vi "Gen Tophat.vi"(1 "Frequency Span":i32=1, 2 "Lower Frequency \nLocation":i32=4, 3 "Nyquist Frequency\nLocation":i32=16) -> (0 "Waveform Graph":i64[](graph))   [LabVIEW 2015]
doc: "This VI will create the actual frequency domain signal required to generate the top hat signal used for acquiring the resonant frequency. The frequency domain signal will be a signal that will span +/- the Nyquist frequency where the waveform is zero at all values except for +/- the frequencies of interest, where the waveform will be one. \n\nThe reflection of the tophat into the negative frequencies ensures that initially we are genrating a sinusoid in the time domain with only a real component (when sampled however, the signal will have both real and imaginary components, but will still have a tophat like structure in the frequency domain). Ultimately, this VI is used to feed into an IDFT for development of a time domain signal."
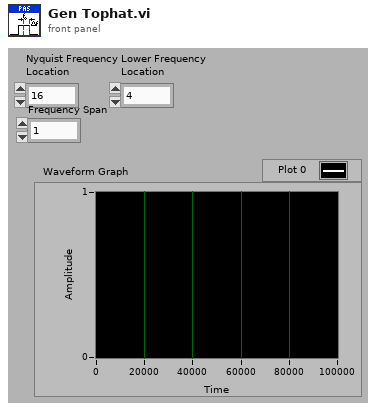
[diagram p1: front panel]
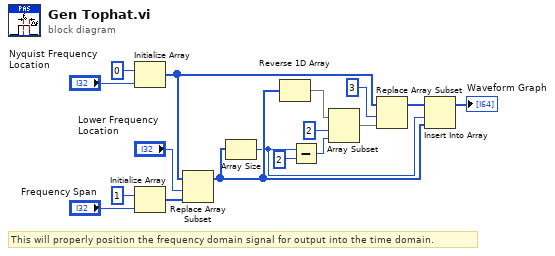
[diagram p0: block diagram]
diagram:
  # "This will properly position the frequency domain signal for output into the time domain."
  n1 = Initialize Array(i64 0 ("element"), "Nyquist Frequency\nLocation") -> (w11:i64[])
  n2 = Initialize Array(i64 1 ("element"), "Frequency Span") -> (w12:i64[])
  n3 = Replace Array Subset(array=w11, new element=w12, index="Lower Frequency \nLocation") -> (w7:i64[])
  n4 = Array Size(array=w7) -> (size(s)=w3:i32)
  n5 = Reverse 1D Array(array=w7) -> (reversed array=w10:i64[])
  n6 = Subtract(x=w3, y=i64 2) -> (x-y=w5:i64)
  n7 = Array Subset(array=w10, index=2, length=w5) -> (w9:i64[])
  n8 = Replace Array Subset(array=w11, new element=w9, index=3) -> (w8:i64[])
  n9 = Insert Into Array(array=w8, index=w3, new element=w7) -> (→"Waveform Graph":i64[])
